vi "Read Haskel.vi"(0 "FPGA API in":refnum<class "FPGA API Concrete.lvclass">, 11 "error in (no error)":errorcluster) -> (4 "FPGA API out":refnum<class "FPGA API Concrete.lvclass">, 6 "Haskel AO Value":dbl, 15 "error out":errorcluster)   [LabVIEW 2019, in "FPGA API Concrete.lvclass"]
uses:
  FPGA API Concrete.lvclass
  FPGA API Concrete.lvclass/FPGA API Concrete.ctl
  <vilib>/Utility/error.llb/Error Cluster From Error Code.vi
  <vilib>/rvi/errors/niLvFpgaAdjustHostInterfaceError.vi
  <vilib>/rvi/interface/nirviReadWriteControl/nirviReadWriteControl.xnode
  FPGA Ref.ctl
  NiFpgaLv.dll
  <vilib>/rvi/interface/Simulation/niFpgaSimulationCallBeginRW.vi
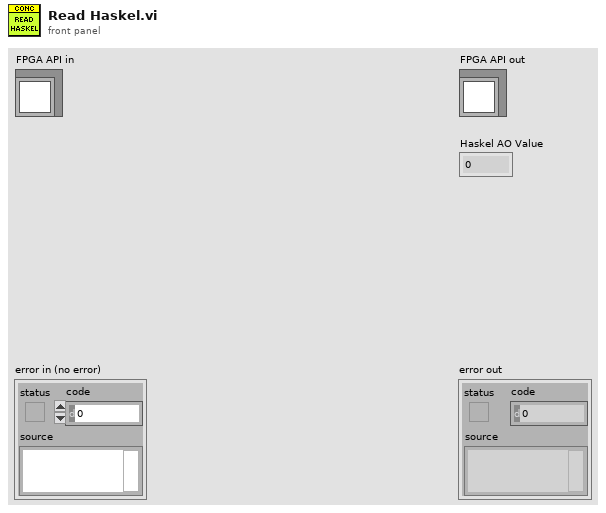
[diagram p1: front panel]
types:
  T1 = typedef "FPGA API Concrete.lvclass/FPGA Ref.ctl" = refnum<k20>
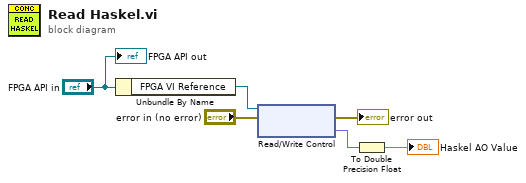
[diagram p0: block diagram]
diagram:
  n1 = Unbundle By Name("FPGA API in") -> ("FPGA VI Reference"=w5:T1)
  n2 = xnode "Read/Write Control"("FPGA VI Reference In"=w5, "error in"="error in (no error)") -> ("error out"=→"error out":errorcluster, "Mod5/AO0"=w2:fxp<+/-,20,5>)  [unwired: 1 out]
  n3 = To Double Precision Float(number=w2) -> (double precision float=→"Haskel AO Value":dbl)
  "FPGA API out" <- "FPGA API in"
